vi "PXI-Config AOAI clk10.vi"(11 "error in (no error)":errorcluster) -> (3 "Sync Task":T1, 4 "AO Tasks":T1[](array[typedef]), 8 "AI Tasks":T1[](array[typedef]), 15 "error out":errorcluster)   [LabVIEW 2020]
uses:
  Type Defs/Task Struct.ctl
  PXI Globals.vi
panel:
  out "Array":dbl[](array[numeric])
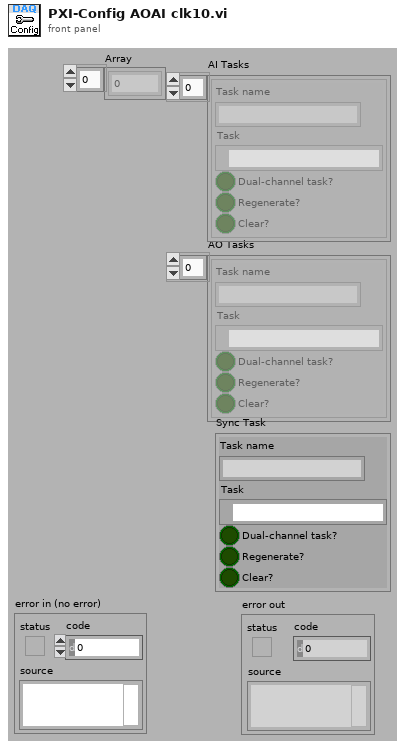
[diagram p1: front panel]
types:
  T1 = typedef "Task Struct.ctl" = cluster{"Task name":string, "Task":refnum<k21>, "Dual-channel task?":bool, "Regenerate?":bool, "Clear?":bool}
  T2 = cluster{"DAQChan to PhysDev":i32[][], "PhysDev to DAQChan":i32[][]}
  T3 = typedef "Channel Struct.ctl" = cluster{"Channel name":string, "Vmax":dbl, "Vmin":dbl, "Rate":dbl, "Terminal configuration":i32, "Physical Channel":tag, "Regenerate":bool}
  T4 = typedef "Task Specification Struct.ctl" = cluster{"Task name":string, "Task":refnum<k21>, "Dual-channel task?":bool, "Channels":T3[]}
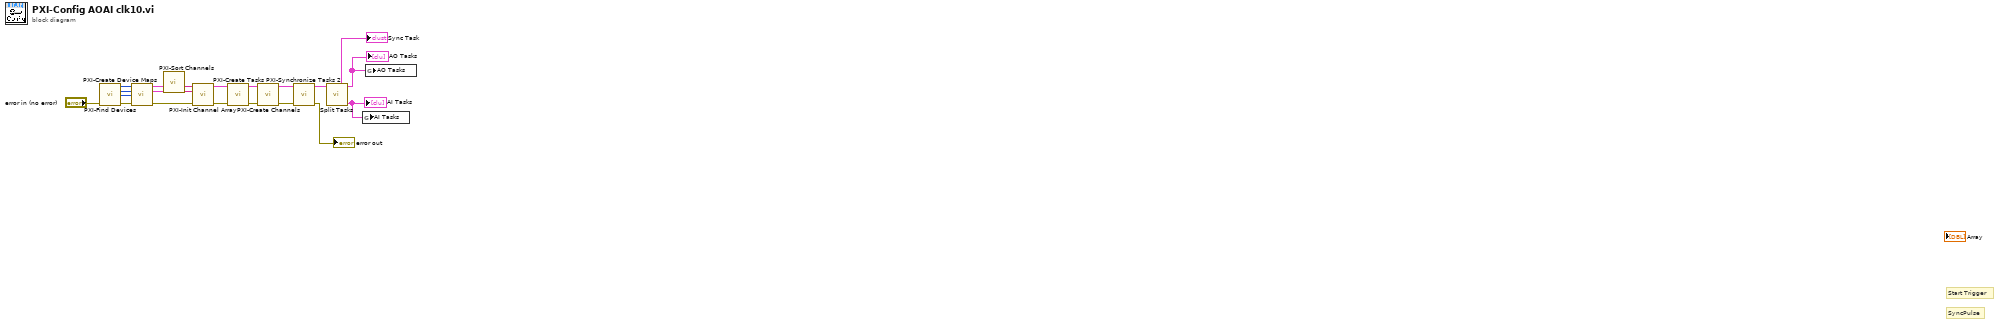
[diagram p0: block diagram]
diagram:
  # "SyncPulse"
  # "Start Trigger"
  n1 = call "PXI-Find Devices.vi"("error in (no error)"="error in (no error)") -> ("Num AO"=w17:i32[], "Num AI"=w16:i32[], "Slot Num"=w19:u32[], "error out"=w18:errorcluster)  [unwired: 11 in]
  n2 = call "PXI-Create Device Maps.vi"("Num AO"=w17, "Num AI"=w16, "Slot Num"=w19, "error in (no error)"=w18) -> ("AO Map"=w15:T2, "AI Map"=w14:T2, "error out"=w13:errorcluster)  [unwired: 9 in]
  n3 = call "PXI-Sort Channels.vi"("AO Map"=w15, "AI Map"=w14) -> ("Sorted channel names"=w10:string[], "Sorted physical channels"=w9:tag[])  [unwired: 12 in]
  n4 = call "PXI-Init Channel Array.vi"("Sorted channel names"=w10, "Sorted physical channels"=w9, "error in (no error)"=w13) -> ("Channel Array"=w11:T3[], "error out"=w12:errorcluster)  [unwired: 11 in]
  n5 = call "PXI-Create Tasks.vi"("I/O Channels"=w11, "error in (no error)"=w12) -> ("Task Specification Array"=w4:T4[], "error out"=w3:errorcluster)  [unwired: 12 in]
  n6 = call "PXI-Create Channels.vi"("Task Specification Array In"=w4, "error in (no error)"=w3) -> ("Task Specification Array Out"=w1:T4[], "error out"=w2:errorcluster)  [unwired: 12 in]
  n7 = call "PXI-Synchronize Tasks 2.vi"("Task Specification Array"=w1, "error in (no error)"=w2) -> ("Task Specification Array Out"=w6:T4[], "error out"=→"error out":errorcluster)  [unwired: 12 in]
  n8 = call "Split Tasks.vi"("Task Specification Array"=w6) -> ("Sync Task"=→"Sync Task":T1, "AO Tasks"=w7:T1[], "AI Tasks"=w8:T1[])  [unwired: 11 in, 1 out]
  "AO Tasks" <- w7
  "AI Tasks" <- w8
  n9 = global write "PXI Globals.vi" "AI Tasks"(w8) -> ()
  n10 = global write "PXI Globals.vi" "AO Tasks"(w7) -> ()
